vi "XSP3_ControlExtraROI.vi"(6 "ExROI":enum16{"Disable", "Enable"}(ring) caption="ControlExtraROI", 8 "ErrorIn":errorcluster, 9 "Ch":i32=1, 11 "ProcessIn":string="XSPRESS3-EXAMPLE" caption="ProcessName") -> (0 "ErrorOut":errorcluster, 2 "Status":bool, 3 "ProcessOut":string caption="ProcessName")   [LabVIEW 2010]
uses:
  Program Files/National Instruments/LabVIEW 2017/user.lib/caLab/Private/Put_I16_PV.vi
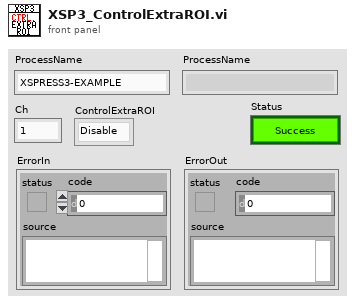
[diagram p1: front panel]
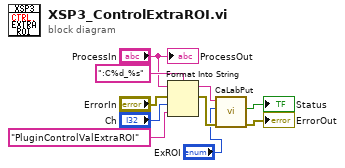
[diagram p0: block diagram]
diagram:
  n1 = Format Into String(format string=":C%d_%s" ("PV"), initial string="ProcessIn", error in="ErrorIn", "Ch", "PluginControlValExtraROI" ("PV")) -> (resulting string=w4:string, error out=w7:errorcluster)
  n2 = call-poly "CaLabPut.vi"("Error in (no error)"=w7, "Value"="ExROI", "PV Name"=w4) -> ("Error out"=→"ErrorOut":errorcluster, "Status"=→"Status":bool)  [unwired: 5 in, 2 out]
  "ProcessOut" <- "ProcessIn"
